vi "Acourse_ConvertDataIn.vi"(8 "error in (no error)":errorcluster, 11 "Cluster in":T1) -> (0 "error out":errorcluster, 2 "Phtr [W]":dbl, 3 "Cluster out":T1)   [LabVIEW 2016]
uses:
  DAQLoop_Typedef.ctl
panel:
  out "Mdot [lbm/h]":dbl
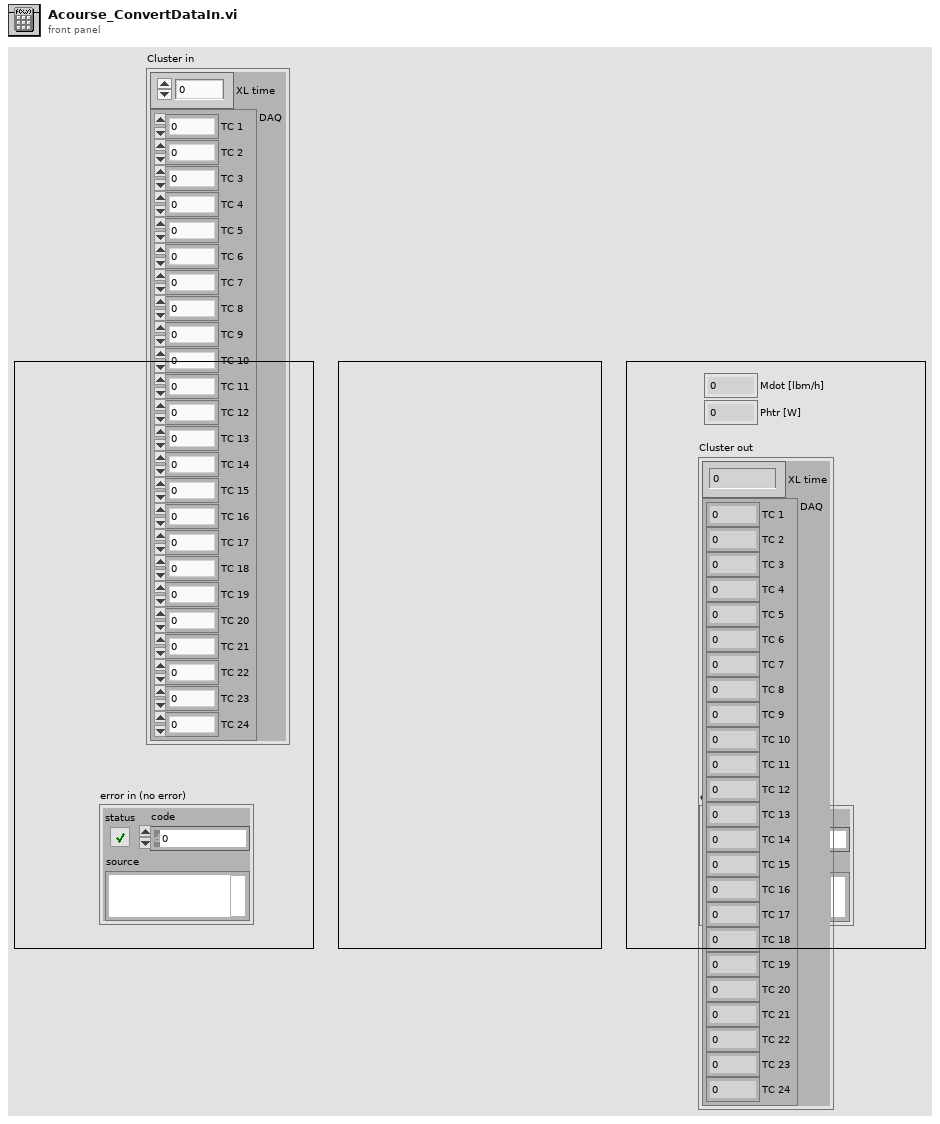
[diagram p1: front panel]
types:
  T1 = typedef "DAQLoop_Typedef.ctl" = cluster{"XL time":dbl, "DAQ":cluster{"TC 1":dbl, "TC 2":dbl, "TC 3":dbl, "TC 4":dbl, "TC 5":dbl, "TC 6":dbl, "TC 7":dbl, "TC 8":dbl, "TC 9":dbl, "TC 10":dbl, "TC 11":dbl, "TC 12":dbl, "TC 13":dbl, "TC 14":dbl, "TC 15":dbl, "TC 16":dbl, "TC 17":dbl, "TC 18":dbl, "TC 19":dbl, "TC 20":dbl, "TC 21":dbl, "TC 22":dbl, "TC 23":dbl, "TC 24":dbl}}
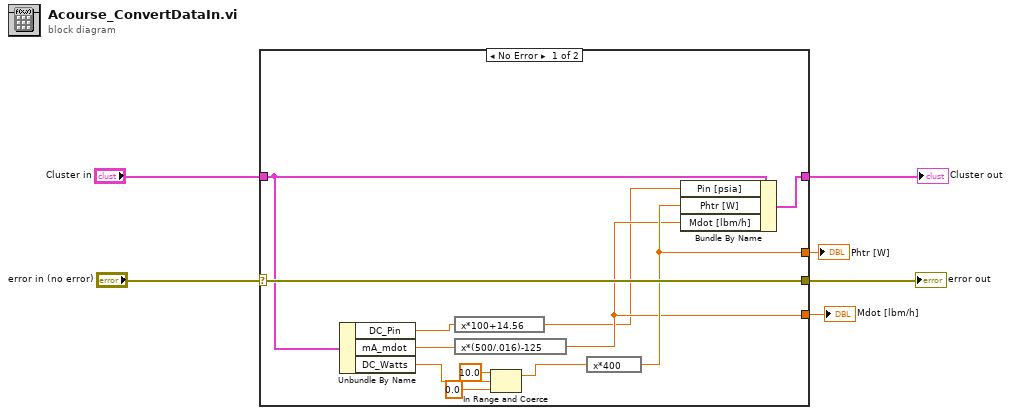
[diagram p0: block diagram]
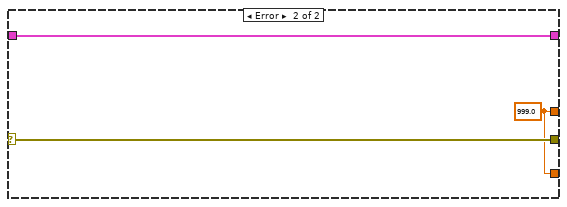
[diagram p2: hidden frame]
diagram:
  n1 = case shown="No Error" "error in (no error)" {
    selector: "error in (no error)" -> [w18 w20]
    tunnel: "Cluster in" -> [w16 w21]
    tunnel: [w15 w21] -> w3
    tunnel: [w18 w20] -> w6
    tunnel: [w13 w19] -> w2
    tunnel: [w12 w19] -> w1
    frame No Error {
      n2 = Unbundle By Name(w16) -> ("DC_Pin"=w8:dbl, "mA_mdot"=w14:dbl, "DC_Watts"=w17:dbl)
      n3 = expression code="x*100+14.56"(w8) -> (w7:dbl)
      n4 = expression code="x*(500/.016)-125"(w14) -> (w12:dbl)
      n5 = In Range and Coerce(upper limit=10.0, x=w17, lower limit=0.0) -> (coerced(x)=w11:dbl)  [unwired: 1 out]
      n6 = expression code="x*400"(w11) -> (w13:dbl)
      n7 = Bundle By Name(cluster=w16, "Pin [psia]"=w7, "Phtr [W]"=w13, "Mdot [lbm/h]"=w12) -> (w15:T1)
    }
    frame Error {
      w19 = 999.0 ("DC_Watts")
    }
  }
  "error out" <- w6
  "Cluster out" <- w3
  "Phtr [W]" <- w2
  "Mdot [lbm/h]" <- w1
